vi "Result.Parse STD OUT Text, Create Result Data_V2.vi"(4 "UUTDir":path, 6 "Prefix":string, 7 "Category":string, 8 "Version Name":string, 9 "Error Code":i32, 10 "Task Name":string, 11 "StdOut":string) -> (0 "Error":errorcluster, 1 "SW Ver":T4[](array[typedef]), 3 "Meas":T2[](array[typedef]) {"Status" items=["LOG", "PASS", "FAIL", "ERROR"]}, 5 "Data Files":T1[](array[typedef]))   [LabVIEW 2018]
uses:
  Result XML/TestResult.SW Item.ctl
  Result.Measurement Item.ctl
  Result.Measurement and Attribute Item Status.ctl
  Reports/Report.Result FileDataObject.ctl
  Errors/Error.Error Code List.ctl
  <vilib>/KATE/Files/File Utils.lvlib
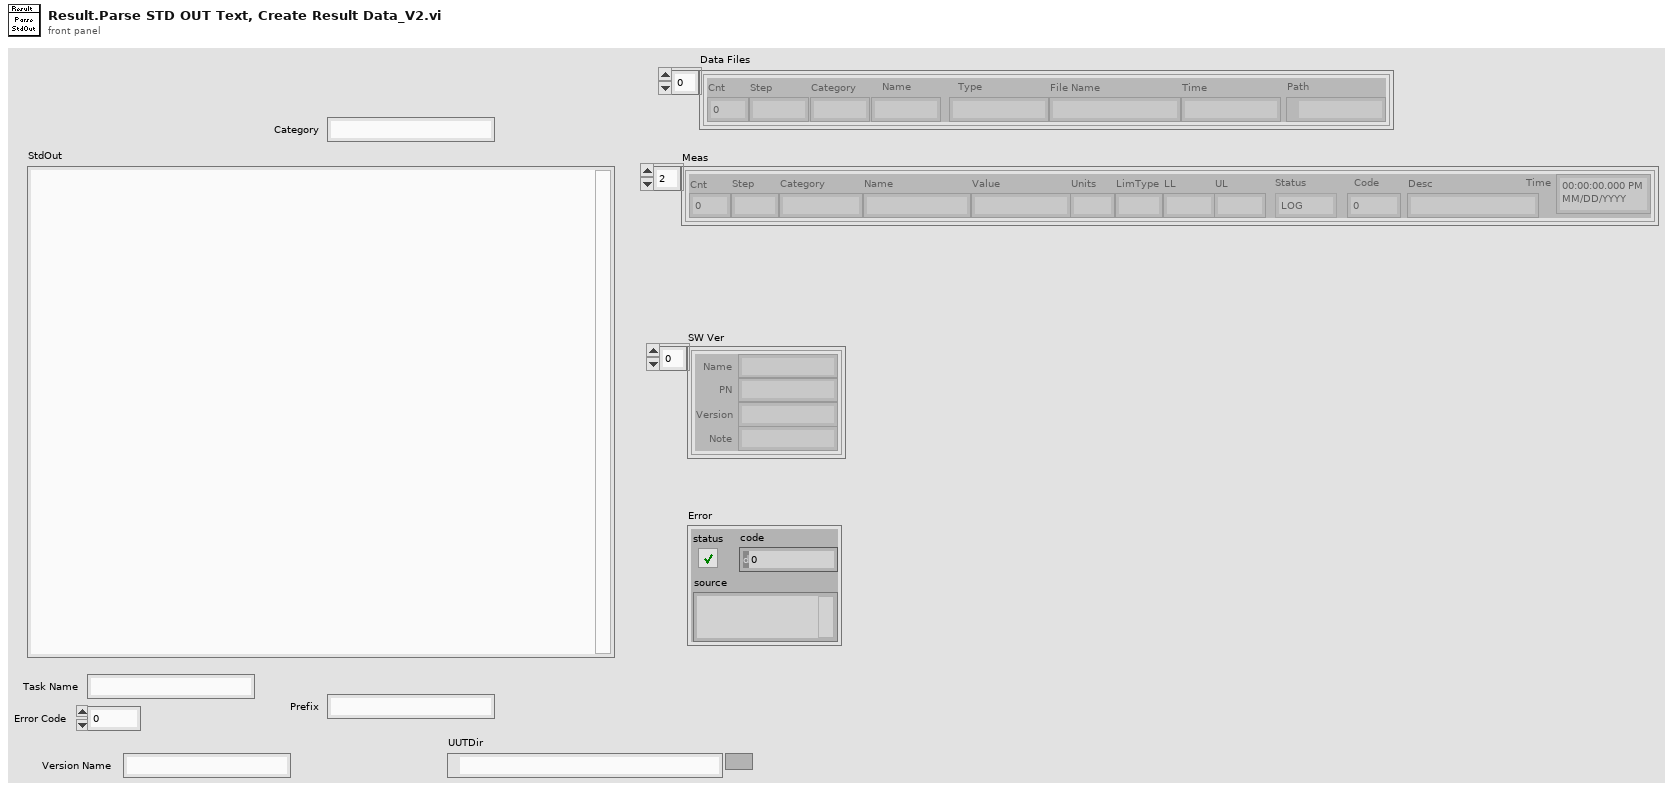
[diagram p1: front panel]
types:
  T1 = typedef "Report.Result FileDataObject.ctl" = cluster{"Cnt":i32, "Step":string, "Category":string, "Name":string, "Type":string, "File Name":string, "Time":string, "Path":path}
  T2 = typedef "Result.Measurement Item.ctl" = cluster{"Cnt":i32, "Step":string, "Category":string, "Name":string, "Value":string, "Units":string, "LimType":string, "LL":string, "UL":string, "Status":T3, "Code":i32, "Desc":string, "Time":timestamp}
  T3 = typedef "Result.Measurement and Attribute Item Status.ctl" = i32
  T4 = typedef "TestResult.SW Item.ctl" = cluster{"Name":string, "PN":string, "Version":string, "Note":string}
  T5 = cluster{"Meas":T2[], "SW Ver":T4[], "Error":errorcluster, "Data Files":T1[]}
  T6 = typedef "Error.Error Code List.ctl" = i32
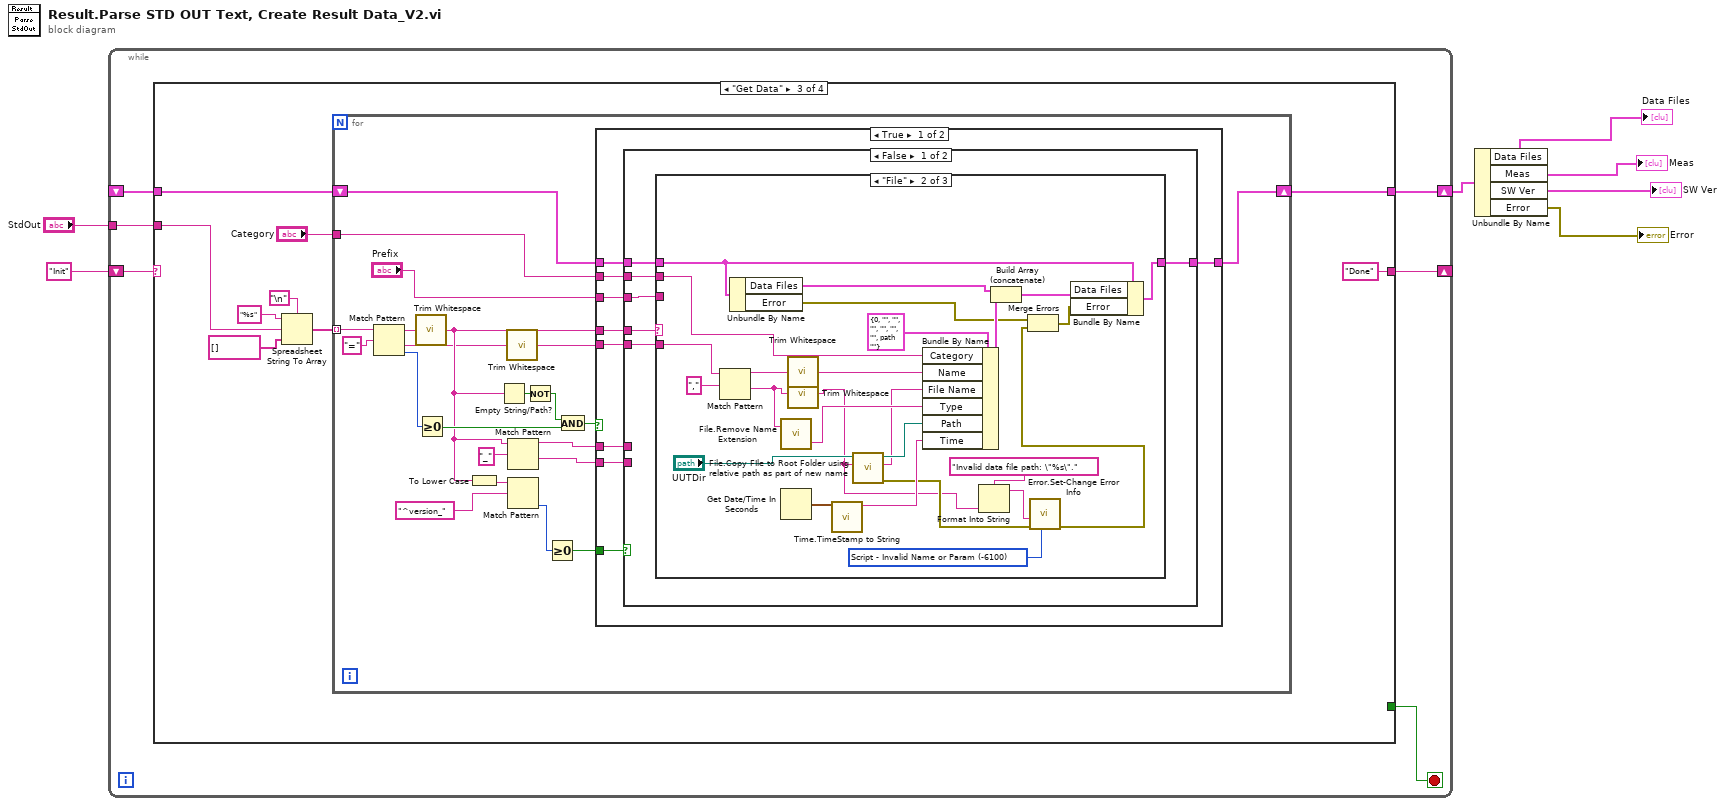
[diagram p0: block diagram]
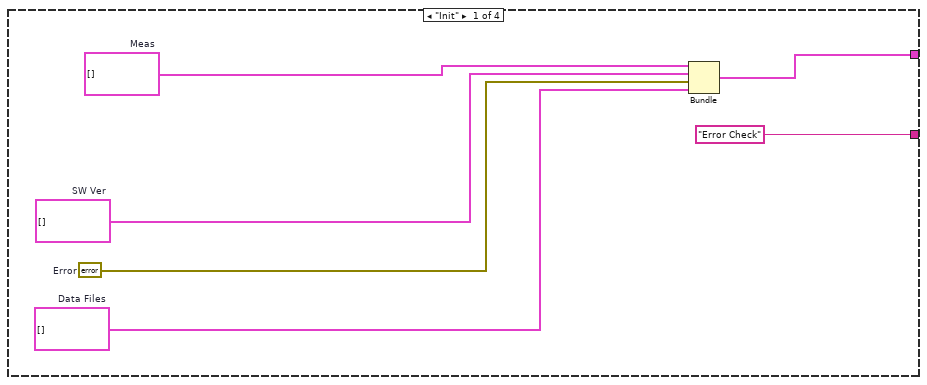
[diagram p2: hidden frame]
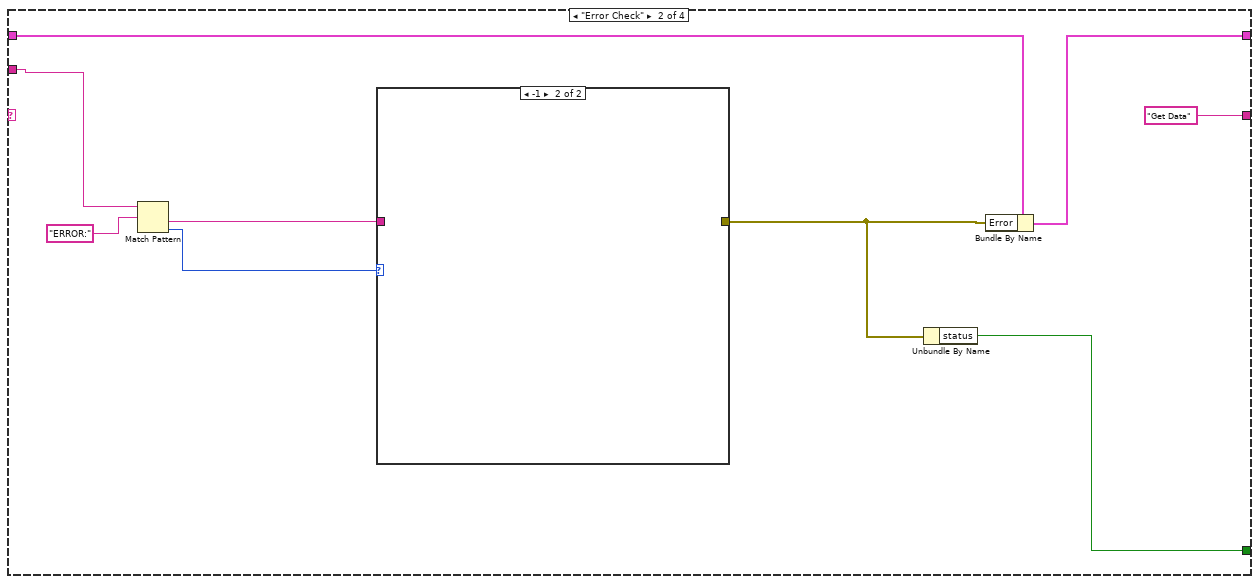
[diagram p3: hidden frame]
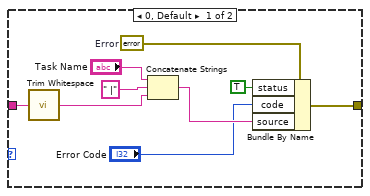
[diagram p4: hidden frame]
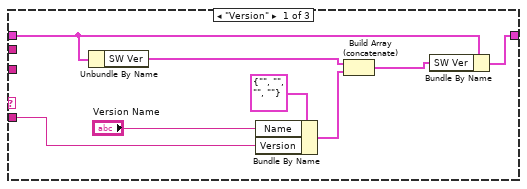
[diagram p5: hidden frame]
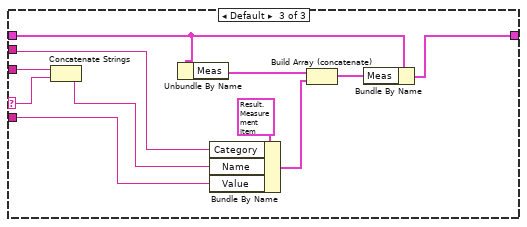
[diagram p6: hidden frame]
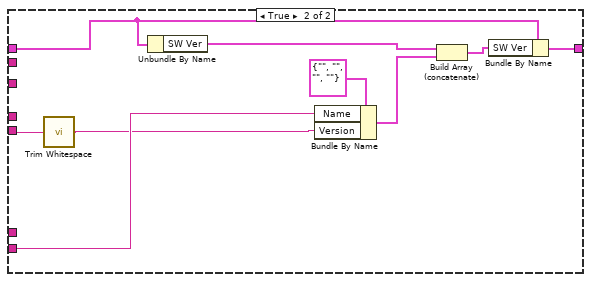
[diagram p7: hidden frame]
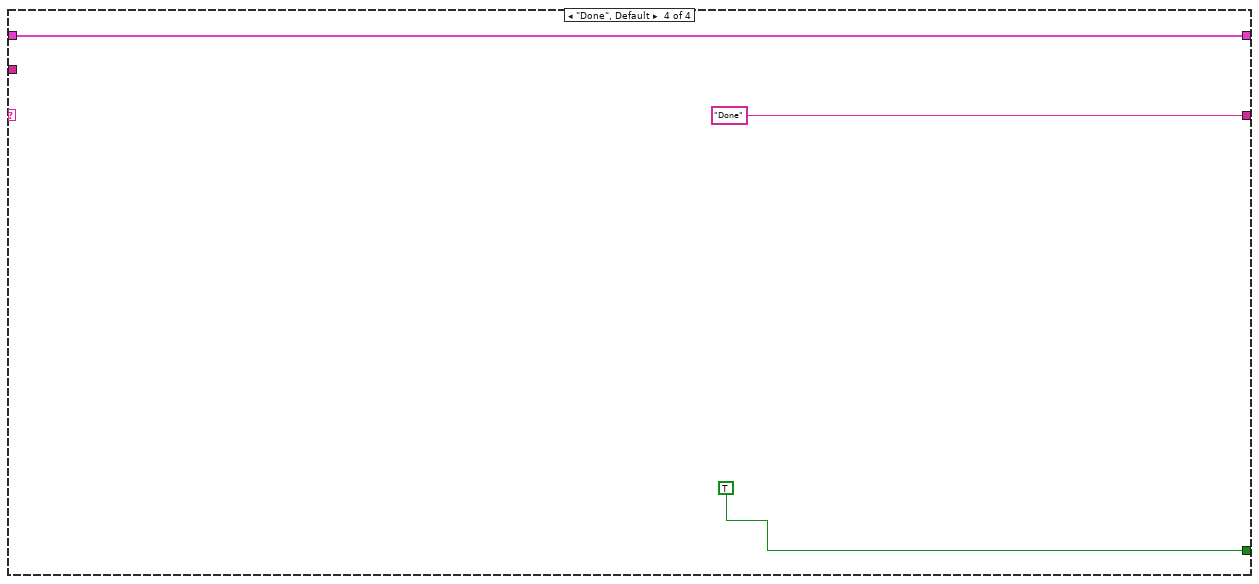
[diagram p9: hidden frame]
diagram:
  n1 = while {
    tunnel: "StdOut" -> [w13]
    shift-right: [w9] -> _
    shift-left: "Init" -> [w12]
    shift-right: [w10] -> w5
    shift-left: _ -> [w11]
    stop <- w8 stop-if-true
    n2 = case shown="\"Get Data\"" w12 {
      tunnel: w13 -> [_ w24 w43 _]
      tunnel: w11 -> [_ w27 w40 w139]
      tunnel: [w17 w26 w38 w139] -> w10
      tunnel: ["Error Check" "Get Data" "Done" "Done"] -> w9
      tunnel: [_ w20 _ TRUE] -> w8
      frame "Init" {
        w14 = T1[] []  # Data Files
        w15 = errorcluster {"status"=FALSE, "code"=0, "source"=""}  # Error
        w19 = T2[] []  # Meas
        w18 = T4[] []  # SW Ver
        n3 = Bundle("Meas"=w19, "SW Ver"=w18, "Error"=w15, "Data Files"=w14) -> (w17:T5)  [unwired: 1 in]
      }
      frame "Error Check" {
        n4 = Match Pattern(string=w24, regular expression="ERROR:") -> (after substring=w23:string, offset past match=w22:i32)  [unwired: 1 in, 2 out]
        n5 = case shown="-1" w22 {
          tunnel: w23 -> [w37 _]
          tunnel: [w29 _] -> w21
          frame 0, Default {
            w36 = errorcluster {"status"=FALSE, "code"=0, "source"=""}  # Error
            n6 = call <vilib>:"Trim Whitespace.vi"("string"=w37) -> ("trimmed string"=w34:string)  [unwired: 1 in]
            n7 = Concatenate Strings("Task Name", " |", w34) -> (w31:string)
            n8 = Bundle By Name(cluster=w36, "status"=TRUE, "code"="Error Code", "source"=w31) -> (w29:errorcluster)
          }
          frame -1 {
          }
        }
        n9 = Unbundle By Name(w21) -> ("status"=w20:bool)
        n10 = Bundle By Name(cluster=w27, "Error"=w21) -> (w26:T5)
      }
      frame "Get Data" {
        n11 = Spreadsheet String To Array(delimiter (Tab)="\n", format string="%s" ("spreadsheet string"), spreadsheet string=w43, array type (2D Dbl)=string[] []) -> (array=w41:string[])
        n12 = for {
          tunnel: w41 -> [w68] mode=indexing
          shift-right: [w65] -> w38
          shift-left: w40 -> [w66]
          tunnel: "Category" -> [w58]
          n13 = Match Pattern(string=w68, regular expression="=") -> (before substring=w64:string, after substring=w48:string, offset past match=w63:i32)  [unwired: 1 in, 1 out]
          n14 = call <vilib>:"Trim Whitespace.vi"("string"=w64) -> ("trimmed string"=w49:string)  [unwired: 1 in]
          n15 = Greater Or Equal To 0?(x=w63) -> (x >= 0?=w60:bool)
          n16 = To Lower Case(string=w49) -> (all lower case string=w53:string)
          n17 = Empty String/Path?(string/path=w49) -> (empty?=w62:bool)
          n18 = call <vilib>:"Trim Whitespace.vi"("string"=w48) -> ("trimmed string"=w47:string)  [unwired: 1 in]
          n19 = Match Pattern(string=w49, regular expression="_") -> (before substring=w52:string, after substring=w51:string)  [unwired: 1 in, 2 out]
          n20 = Match Pattern(string=w53, regular expression="^version_") -> (offset past match=w56:i32)  [unwired: 1 in, 3 out]
          n21 = Not(x=w62) -> (.not. x?=w61:bool)
          n22 = Greater Or Equal To 0?(x=w56) -> (x >= 0?=w55:bool)
          n23 = And(x=w61, y=w60) -> (x .and. y?=w59:bool)
          n24 = case shown="True" w59 {
            tunnel: w66 -> [w75 w138]
            tunnel: [w74 w138] -> w65
            tunnel: w47 -> [w77 _]
            tunnel: w49 -> [w73 _]
            tunnel: w58 -> [w76 _]
            tunnel: "Prefix" -> [w72 _]
            tunnel: w52 -> [w69 _]
            tunnel: w51 -> [w70 _]
            tunnel: w55 -> [w71 _]
            frame True {
              n25 = case shown="False" w71 {
                tunnel: w77 -> [w83 w130]
                tunnel: w76 -> [w82 _]
                tunnel: w75 -> [w81 w132]
                tunnel: [w80 w133] -> w74
                tunnel: w73 -> [w79 _]
                tunnel: w72 -> [w78 _]
                tunnel: w70 -> [_ w131]
                tunnel: w69 -> [_ _]
                frame False {
                  n26 = case shown="\"File\"" w79 {
                    selector: w79 -> [_ _ w123]
                    tunnel: w83 -> [w84 w104 w128]
                    tunnel: w82 -> [_ w111 w124]
                    tunnel: w81 -> [w90 w100 w127]
                    tunnel: [w89 w117 w126] -> w80
                    tunnel: w78 -> [_ _ w125]
                    frame "Version" {
                      n27 = Unbundle By Name(w90) -> ("SW Ver"=w87:T4[])
                      n28 = Bundle By Name(cluster=T4 {"Name"="", "PN"="", "Version"="", "Note"=""} ("SW_Item"), "Name"="Version Name", "Version"=w84) -> (w86:T4)
                      n29 = Build Array (concatenate)(w87, w86) -> (w88:T4[])
                      n30 = Bundle By Name(cluster=w90, "SW Ver"=w88) -> (w89:T5)
                    }
                    frame "File" {
                      w96 = T6 -6100 items=["No Error"=0, "Abort"=-2, "Misc"=-5000, "Fixture Error"=-5100, "File IO - General"=-5200, "FIle IO - Config Error"=-5201, "Instrument - General"=-5300, "Instrument - Serial Com"=-5301, "Instrument - Camera"=-5302, "Instrument - PS"=-5303, "Instrument - Oscilloscope"=-5304, "Instrument - Function Gen"=-5305, "Instrument - Load"=-5306, "Instrument - Meter"=-5307, "Instrument - Power Control"=-5308, "Instrument - Motion"=-5309, "Instrument - RF"=-5310, "System Exe"=-5400, "Image Processing"=-5500, "Communication"=-5600, "Script - Syntax Error"=-6000, "Script - Invalid Name or Param"=-6100, "Script - Timeout"=-6200, "Invalid Data"=-6300, "FW Update Error"=-6500] ("Std Code")
                      n31 = Match Pattern(string=w104, regular expression=",") -> (before substring=w109:string, after substring=w107:string)  [unwired: 1 in, 2 out]
                      n32 = Unbundle By Name(w100) -> ("Data Files"=w115:T1[], "Error"=w98:errorcluster)
                      n33 = call <vilib>:"File.Remove Name Extension.vi"("File Name"=w107) -> ("Ext"=w108:string)  [unwired: 1 in, 1 out]
                      n34 = Get Date/Time In Seconds() -> (seconds since 1Jan1904=w106:timestamp)
                      n35 = call <vilib>:"Trim Whitespace.vi"("string"=w109) -> ("trimmed string"=w110:string)  [unwired: 1 in]
                      n36 = call <vilib>:"Trim Whitespace.vi"("string"=w107) -> ("trimmed string"=w93:string)  [unwired: 1 in]
                      n37 = call "Time.TimeStamp to String.vi"("Time Stamp in"=w106) -> ("Time String Out"=w105:string)  [unwired: 10 in]
                      n38 = call "File.Copy FIle to Root Folder using relative path as part of new name.vi"("Relative Path"=w93, "Root Path"="UUTDir") -> ("error out"=w97:errorcluster, "New File Name"=w101:string, "Adjusted Path"=w102:path)  [unwired: 6 in, 1 out]
                      n39 = Bundle By Name(cluster=T1 {"Cnt"=0, "Step"="", "Category"="", "Name"="", "Type"="", "File Name"="", "Time"="", "Path"=path ""} ("FileData Object"), "Category"=w111, "Name"=w110, "File Name"=w101, "Type"=w108, "Path"=w102, "Time"=w105) -> (w114:T1)
                      n40 = Format Into String(format string="Invalid data file path: \"%s\".", w93) -> (resulting string=w94:string)  [unwired: 2 in, 1 out]
                      n41 = Build Array (concatenate)(w115, w114) -> (w116:T1[])
                      n42 = call "Error.Set-Change Error Info.vi"("Std Code"=w96, "error in"=w97, "Description"=w94) -> ("error out"=w92:errorcluster)  [unwired: 8 in]
                      n43 = Merge Errors(w98, w92) -> (w99:errorcluster)
                      n44 = Bundle By Name(cluster=w100, "Data Files"=w116, "Error"=w99) -> (w117:T5)
                    }
                    frame Default {
                      n45 = Concatenate Strings(w125, w123) -> (w122:string)
                      n46 = Unbundle By Name(w127) -> ("Meas"=w120:T2[])
                      n47 = Bundle By Name(cluster=T2 {"Cnt"=0, "Step"="", "Category"="", "Name"="", "Value"="", "Units"="", "LimType"="", "LL"="", "UL"="", "Status"=0, "Code"=0, "Desc"="", "Time"=timestamp(0 s since 1904-01-01)} ("Meas"), "Category"=w124, "Name"=w122, "Value"=w128) -> (w119:T2)
                      n48 = Build Array (concatenate)(w120, w119) -> (w118:T2[])
                      n49 = Bundle By Name(cluster=w127, "Meas"=w118) -> (w126:T5)
                    }
                  }
                }
                frame True {
                  n50 = call <vilib>:"Trim Whitespace.vi"("string"=w130) -> ("trimmed string"=w129:string)  [unwired: 1 in]
                  n51 = Unbundle By Name(w132) -> ("SW Ver"=w135:T4[])
                  n52 = Bundle By Name(cluster=T4 {"Name"="", "PN"="", "Version"="", "Note"=""} ("SW_Item"), "Name"=w131, "Version"=w129) -> (w134:T4)
                  n53 = Build Array (concatenate)(w135, w134) -> (w136:T4[])
                  n54 = Bundle By Name(cluster=w132, "SW Ver"=w136) -> (w133:T5)
                }
              }
            }
            frame False {
            }
          }
        }
      }
      frame "Done", Default {
      }
    }
  }
  n55 = Unbundle By Name(w5) -> ("Data Files"=→"Data Files":T1[], "Meas"=→"Meas":T2[], "SW Ver"=→"SW Ver":T4[], "Error"=→"Error":errorcluster)
